vi "UsrProfiles-Previous session.vi"(8 "error in (no error)":errorcluster) -> (0 "error out":errorcluster, 3 "Previous session profile selected":bool)   [LabVIEW 2017]
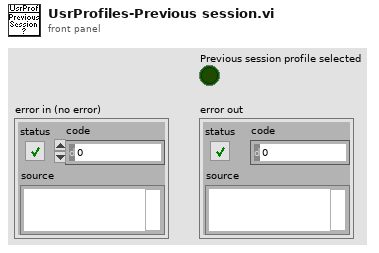
[diagram p1: front panel]
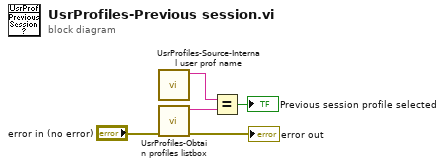
[diagram p0: block diagram]
diagram:
  n1 = call "UsrProfiles-Source-Internal user prof name.vi"() -> ("Previous session profile name"=w2:string)  [unwired: 11 in]
  n2 = call "UsrProfiles-Obtain profiles listbox.vi"("error in (no error)"="error in (no error)") -> ("error out"=→"error out":errorcluster, "Selected profile's name"=w4:string)  [unwired: 7 in, 2 out]
  n3 = Equal?(x=w2, y=w4) -> (x = y?=→"Previous session profile selected":bool)
